vi "Get Capabilities.vi"(0 "object in":refnum<class "HPS-17000-PowerModule.lvclass">, 11 "Error In":errorcluster) -> (4 "object out":refnum<class "HPS-17000-PowerModule.lvclass">, 6 "modes":string[](array[string]), 8 "ranges":string[](array[string]), 15 "Error Out":errorcluster)   [LabVIEW 2023, in "HPS-17000-PowerModule.lvlib" / "HPS-17000-PowerModule.lvclass"]
uses:
  HPS-17000-PowerModule.lvclass
  HPS-17000-PowerModule.lvclass/HPS-17000-PowerModule.ctl
  Mode.ctl
  Range.ctl
panel:
  in  "RANGE":T1 items=["0,750 V / -480,480 A", "0,1500 V / -240,240 A"]
  in  "MODE":T2=193 items=["NULL"=0, "CONSTANT VOLTAGE (V+R)"=1, "CONSTANT CURRENT (I)"=2, "V_VCC"=33, "V_VCC_R"=34, "V_VCC_RADJ"=35, "V_PI_IINT"=177, "INTERNAL RECIRCULATION (VCC)"=193, "INTERNAL RECIRCULATION (B2B)"=209, "VOLTAGE REFORMATION"=225]
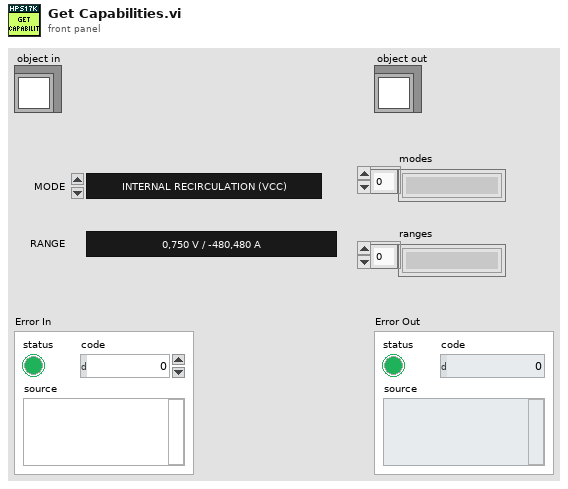
[diagram p1: front panel]
types:
  T1 = typedef "HPS-17000-PowerModule.lvlib/HPS-17000-PowerModule.lvclass/Range.ctl" = u16
  T2 = typedef "HPS-17000-PowerModule.lvlib/HPS-17000-PowerModule.lvclass/Mode.ctl" = u16
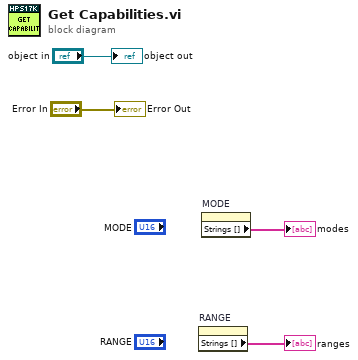
[diagram p0: block diagram]
diagram:
  n1 = property on="RANGE" class="Ring (strict)"() -> ("Strings []"=→"ranges":string[])  [unwired: 2 in, 2 out]
  n2 = property on="MODE" class="Ring (strict)"() -> ("Strings []"=→"modes":string[])  [unwired: 2 in, 2 out]
  "Error Out" <- "Error In"
  "object out" <- "object in"
